vi "client_chat.vi"(1 "port":u16, 2 "address":string) -> (0 "queue out":refnum<queue>)   [LabVIEW 2024]
panel:
  in  "send":bool
  in  "String 2":string
  in  "stop":bool
  out "String":string
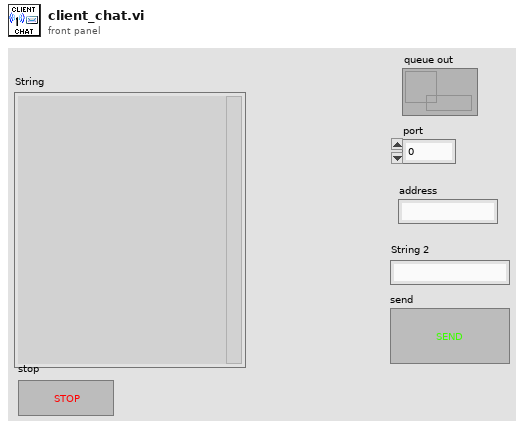
[diagram p1: front panel]
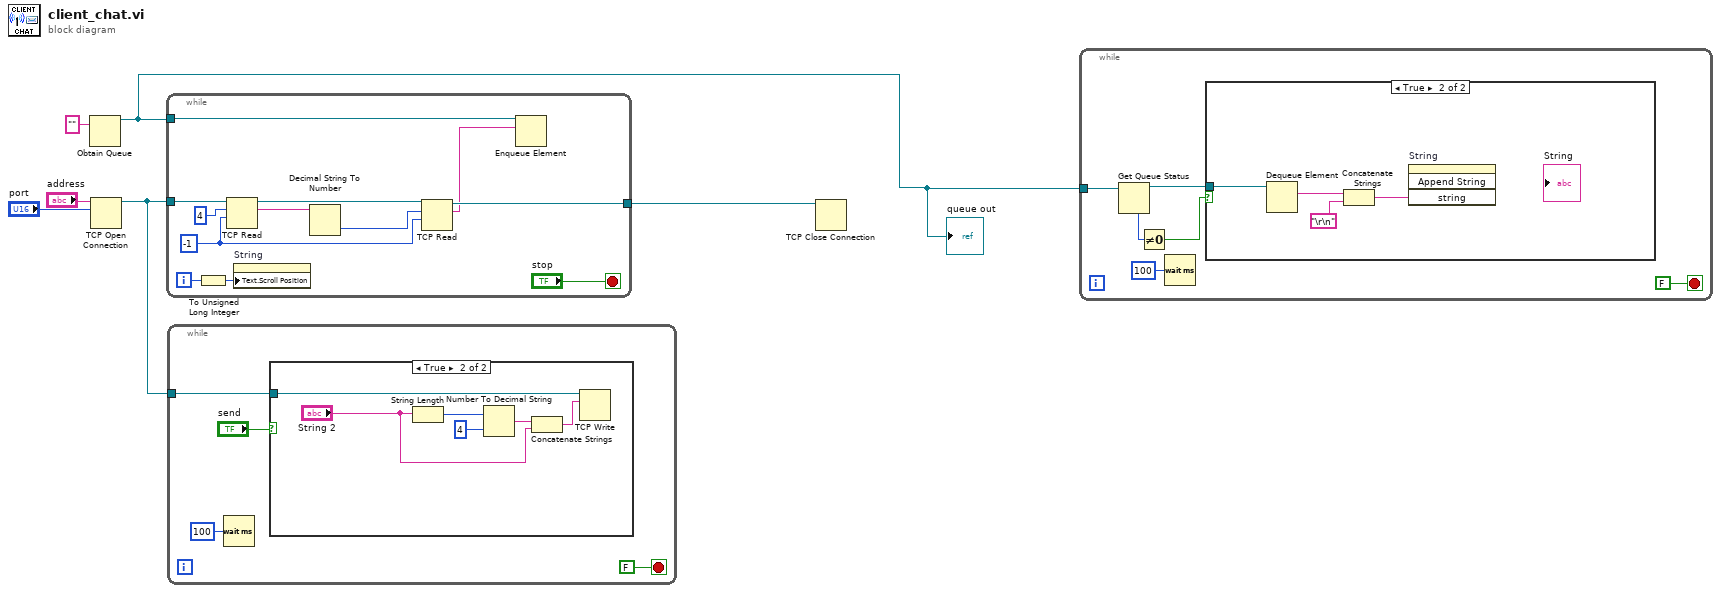
[diagram p0: block diagram]
diagram:
  n1 = Obtain Queue(element data type="") -> (queue out=w5:refnum<queue>)  [unwired: 4 in, 2 out]
  "queue out" <- w5
  n2 = TCP Open Connection(address="address", remote port or service name="port") -> (connection ID=w1:refnum<k5>)  [unwired: 1 in, 3 out]
  n3 = while {
    tunnel: w1 -> [w15]
    tunnel: [w18] -> w6
    tunnel: w5 -> [w7]
    i -> [w9]
    stop <- "stop" stop-if-true
    w16 = -1 ("timeout ms (25000)")
    n4 = To Unsigned Long Integer(number=w9) -> (unsigned 32bit integer=w10:u32)
    n5 = TCP Read(connection ID=w15, bytes to read=4, 9:w16) -> (connection ID out=w13:refnum<k5>, data out=w12:string)  [unwired: 1 in, 2 out]
    n6 = property on="String" class="Str"("Text.Scroll Position"=w10) -> ()  [unwired: 2 in, 2 out]
    n7 = Decimal String To Number(string=w12) -> (number=w11:i32)  [unwired: 2 in, 1 out]
    n8 = TCP Read(connection ID=w13, bytes to read=w11, 9:w16) -> (connection ID out=w18:refnum<k5>, data out=w8:string)  [unwired: 1 in, 2 out]
    n9 = Enqueue Element(queue=w7, element=w8) -> ()  [unwired: 2 in, 3 out]
  }
  n10 = while {
    tunnel: w1 -> [w19]
    stop <- FALSE stop-if-true
    n11 = Wait (ms)(milliseconds to wait=u32 100) -> ()  [unwired: 1 out]
    n12 = case shown="True" "send" {
      tunnel: w19 -> [_ w23]
      frame False {
      }
      frame True {
        n13 = String Length(string="String 2") -> (length=w26:i32)
        n14 = Number To Decimal String(number=w26, width (-)=i16 4) -> (decimal integer string=w28:string)
        n15 = Concatenate Strings(w28, "String 2") -> (w27:string)
        n16 = TCP Write(connection ID=w23, data in=w27) -> ()  [unwired: 2 in, 3 out]
      }
    }
  }
  n17 = TCP Close Connection(connection ID=w6) -> ()  [unwired: 1 in, 3 out]
  n18 = while {
    tunnel: w5 -> [w31]
    stop <- FALSE stop-if-true
    n19 = Get Queue Status(queue=w31) -> (queue out=w30:refnum<queue>, # elements in queue=w33:i32)  [unwired: 2 in, 6 out]
    n20 = Not Equal To 0?(x=w33) -> (x != 0?=w32:bool)
    n21 = Wait (ms)(milliseconds to wait=u32 100) -> ()  [unwired: 1 out]
    n22 = case shown="True" w32 {
      tunnel: w30 -> [_ w38]
      frame False {
      }
      frame True {
        n23 = Dequeue Element(queue=w38) -> (element=w35:string)  [unwired: 2 in, 3 out]
        n24 = Concatenate Strings(w35, "\r\n") -> (w36:string)
        n25 = invoke on="String" class="Str" method="Append String"("string"=w36) -> ()  [unwired: 3 in, 4 out]
      }
    }
  }
